vi "quiz3_valecopia.vi"() -> ()   [LabVIEW 2017]
panel:
  out "Usuarios Existentes 2":string[][](array[string])
  out "Leer 2":string[][](array[string])
  out "array 2":string[][](array[string])
  out "Tamaño users 2":i32
  out "Tab Control 2":enum32{"Page 1", "Page 2", "Page 3"}(tab)
  in  "Ingresar 2":bool
  in  "Usuario 2":string
  in  "Contraseña  2":string
  in  "Regresar 3":bool
  in  "ver usuarios 2":bool
  in  "Borrar usuario 2":string
  in  "Eliminar 2":bool
  in  "Agregar 2":bool
  in  "Contraseña usuario 2":string
  in  "nuevo usuario 2":string
  in  "Regresar 4":bool
  out "Leer":string[][](array[string])
  out "Usuarios Existentes":string[][](array[string])
  out "Tamaño users":i32
  out "array":string[][](array[string])
  out "Tab Control":enum32{"Page 1", "Page 2", "Page 3"}(tab)
  in  "Ingresar":bool
  in  "Usuario":string
  in  "Contraseña":string
  in  "Regresar":bool
  in  "ver usuarios":bool
  in  "Borrar usuario":string
  in  "Eliminar":bool
  in  "Agregar":bool
  in  "Contraseña usuario":string
  in  "nuevo usuario":string
  in  "Regresar 2":bool
  # "HOLIII..!"
  # "HOLIII..!"
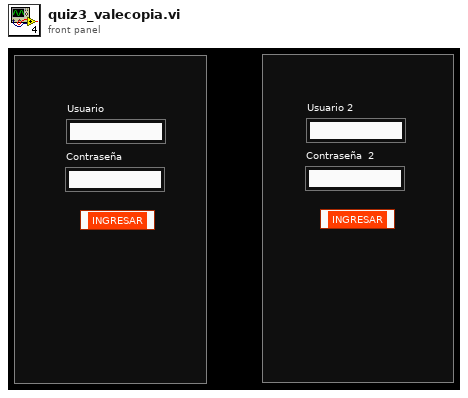
[diagram p1: front panel]
types:
  T1 = enum16{"open", "replace", "create", "open or create", "replace or create", "replace or create with confirmation"}
  T2 = typedef "Semaphore RefNum" = refnum<k1>
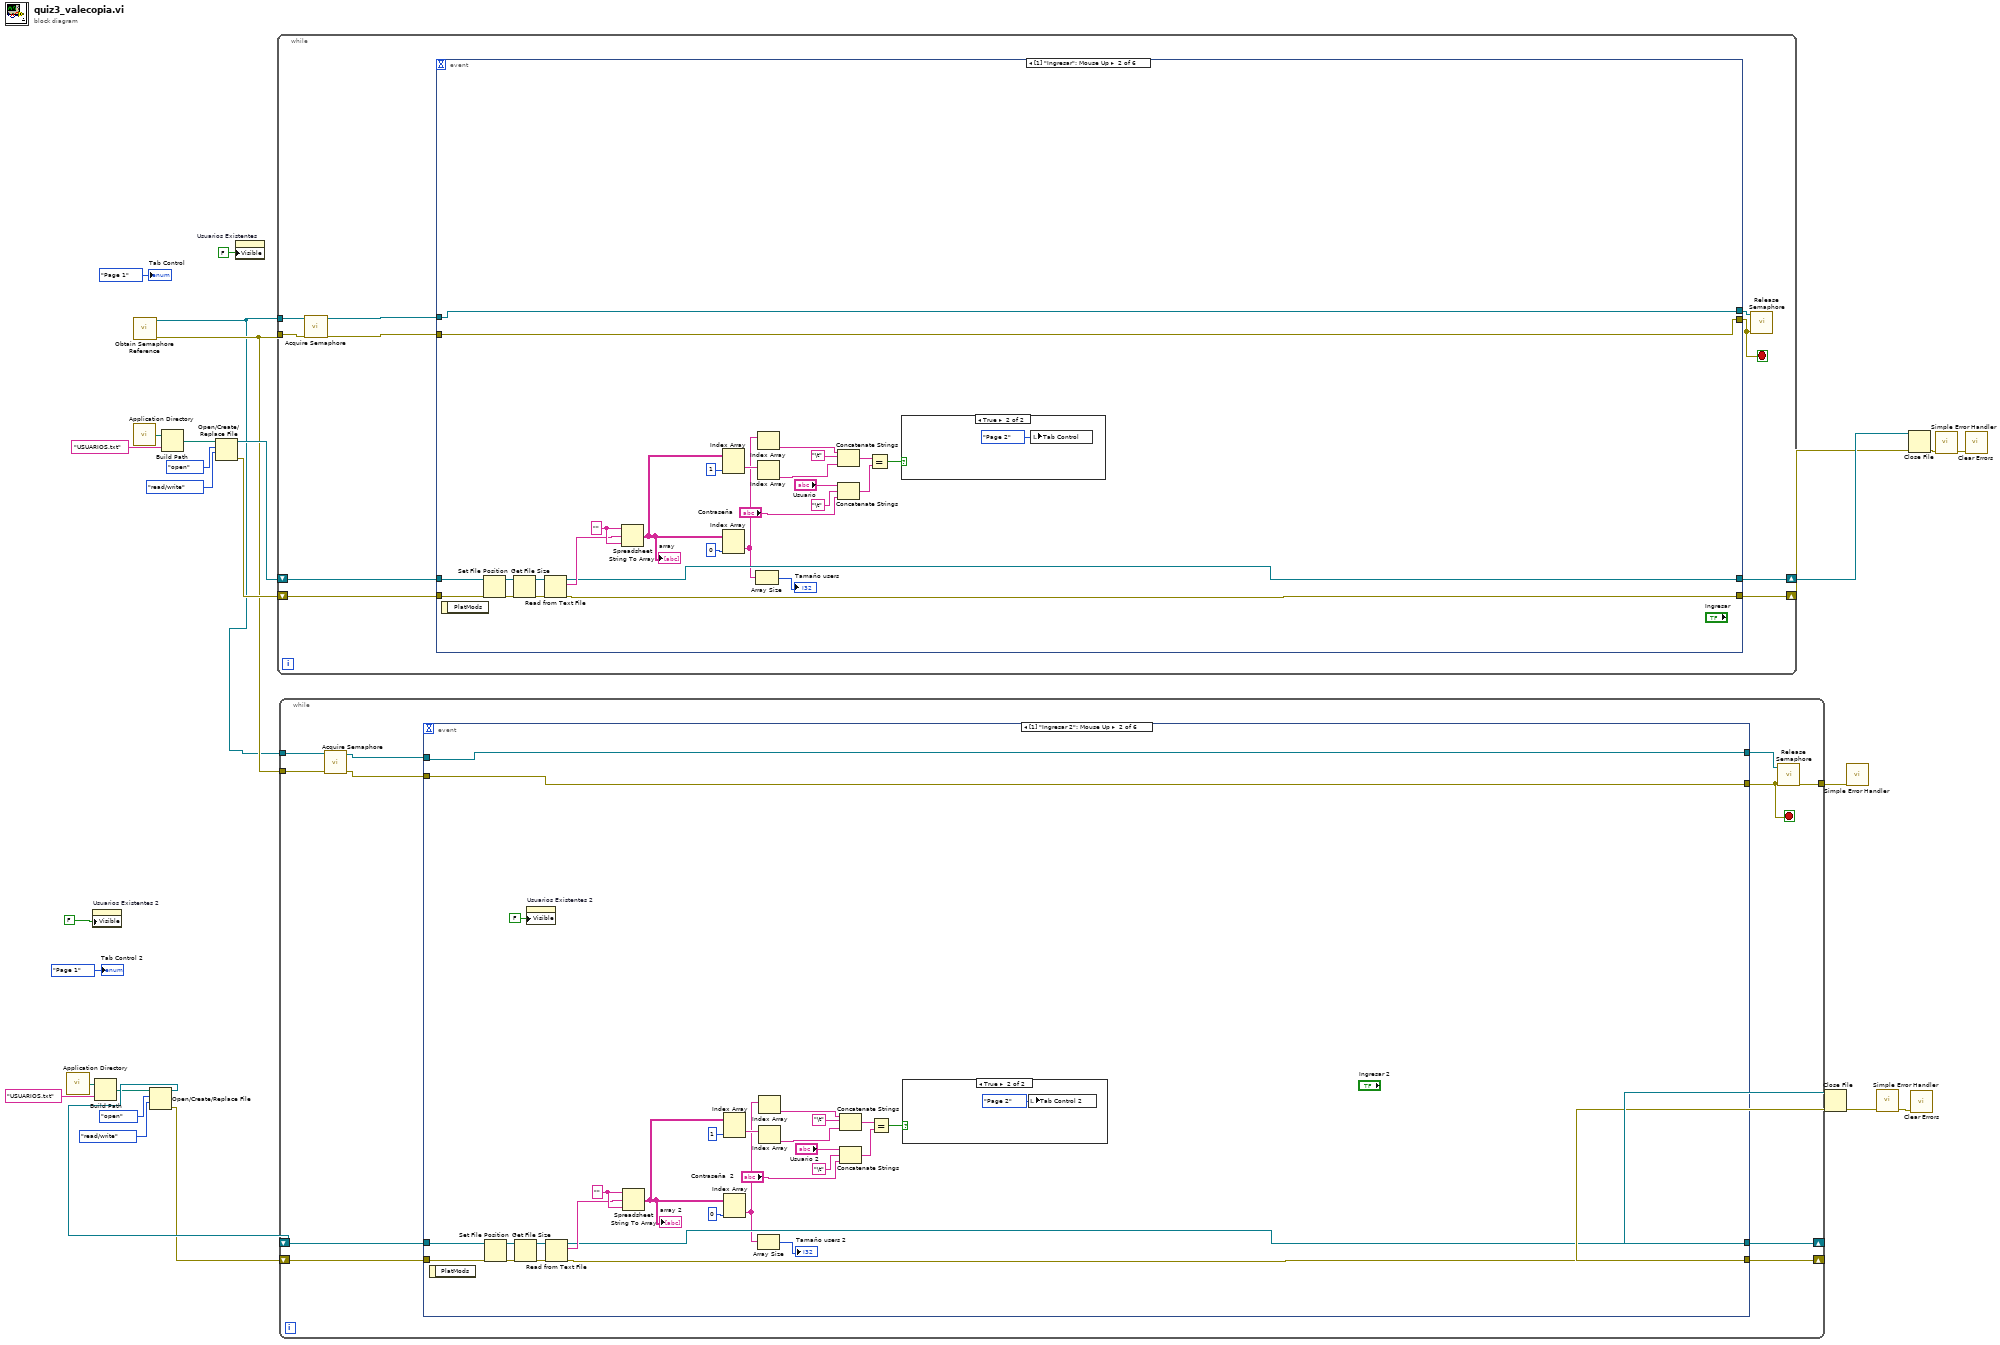
[diagram p0: block diagram]
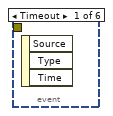
[diagram p2: hidden frame]
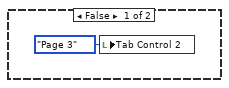
[diagram p3: hidden frame]
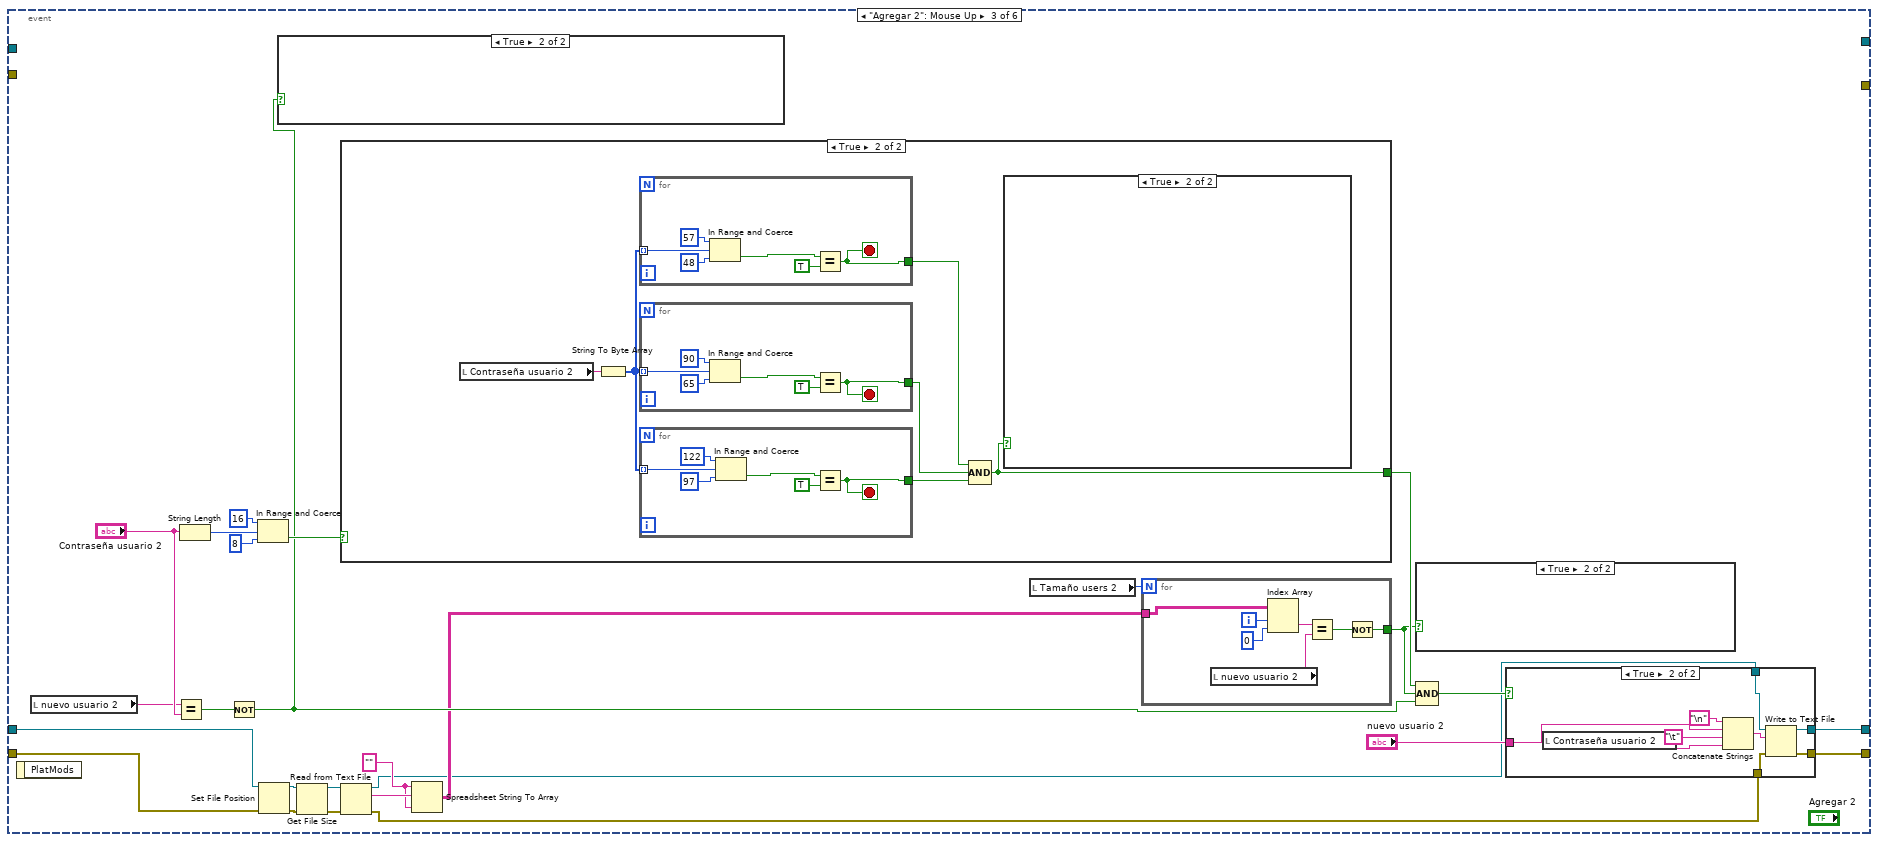
[diagram p4: hidden frame]
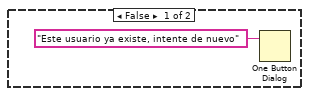
[diagram p5: hidden frame]
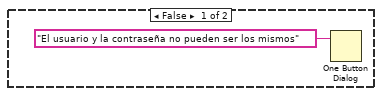
[diagram p6: hidden frame]
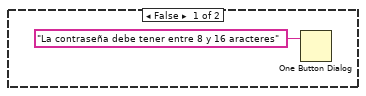
[diagram p8: hidden frame]
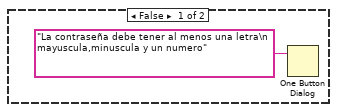
[diagram p9: hidden frame]
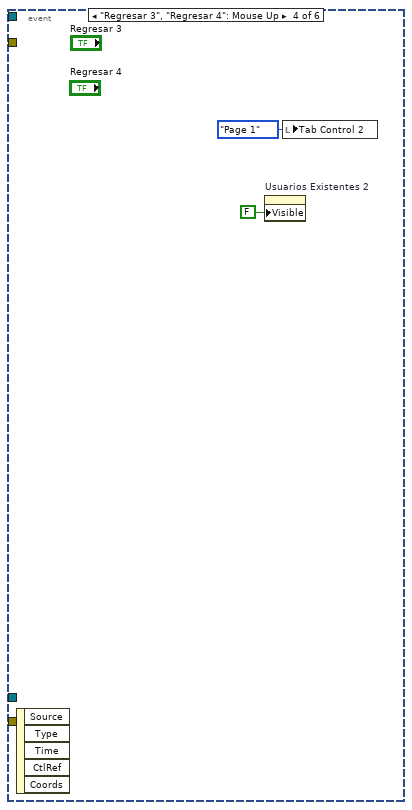
[diagram p10: hidden frame]
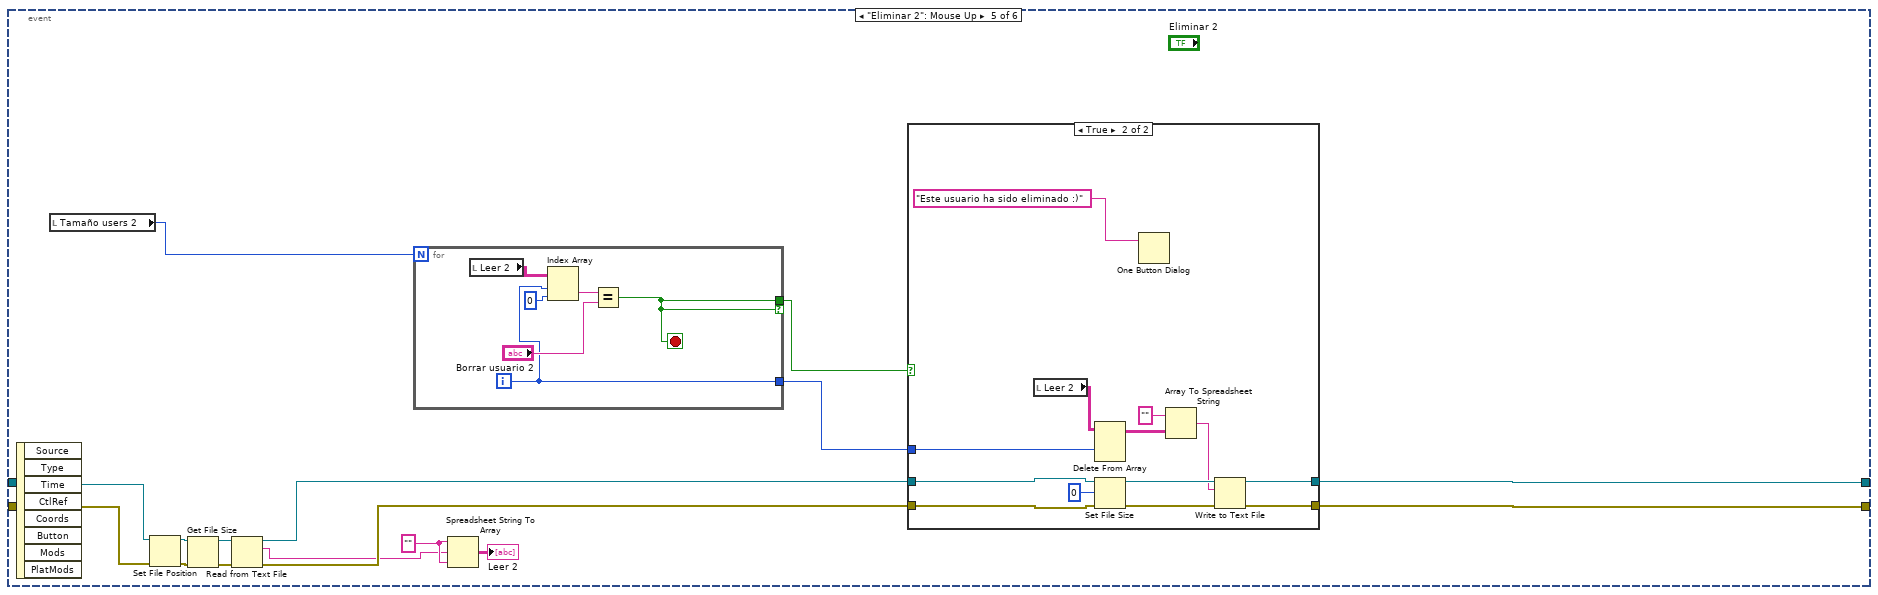
[diagram p11: hidden frame]
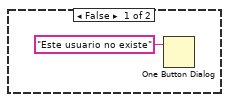
[diagram p12: hidden frame]
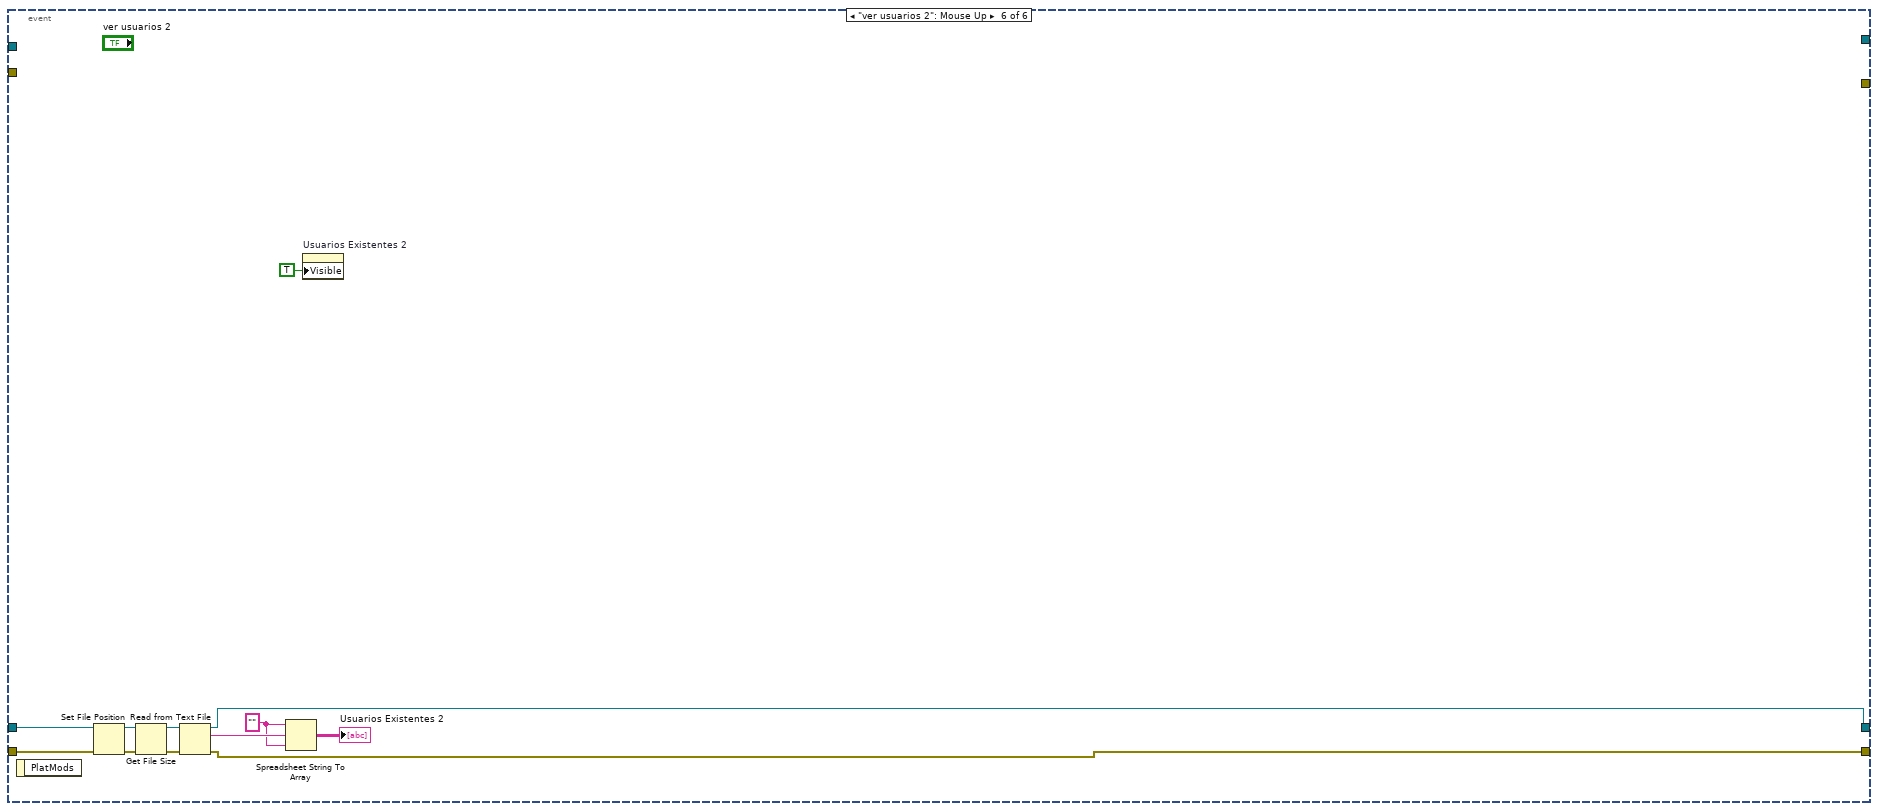
[diagram p13: hidden frame]
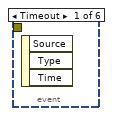
[diagram p14: hidden frame]
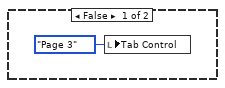
[diagram p15: hidden frame]
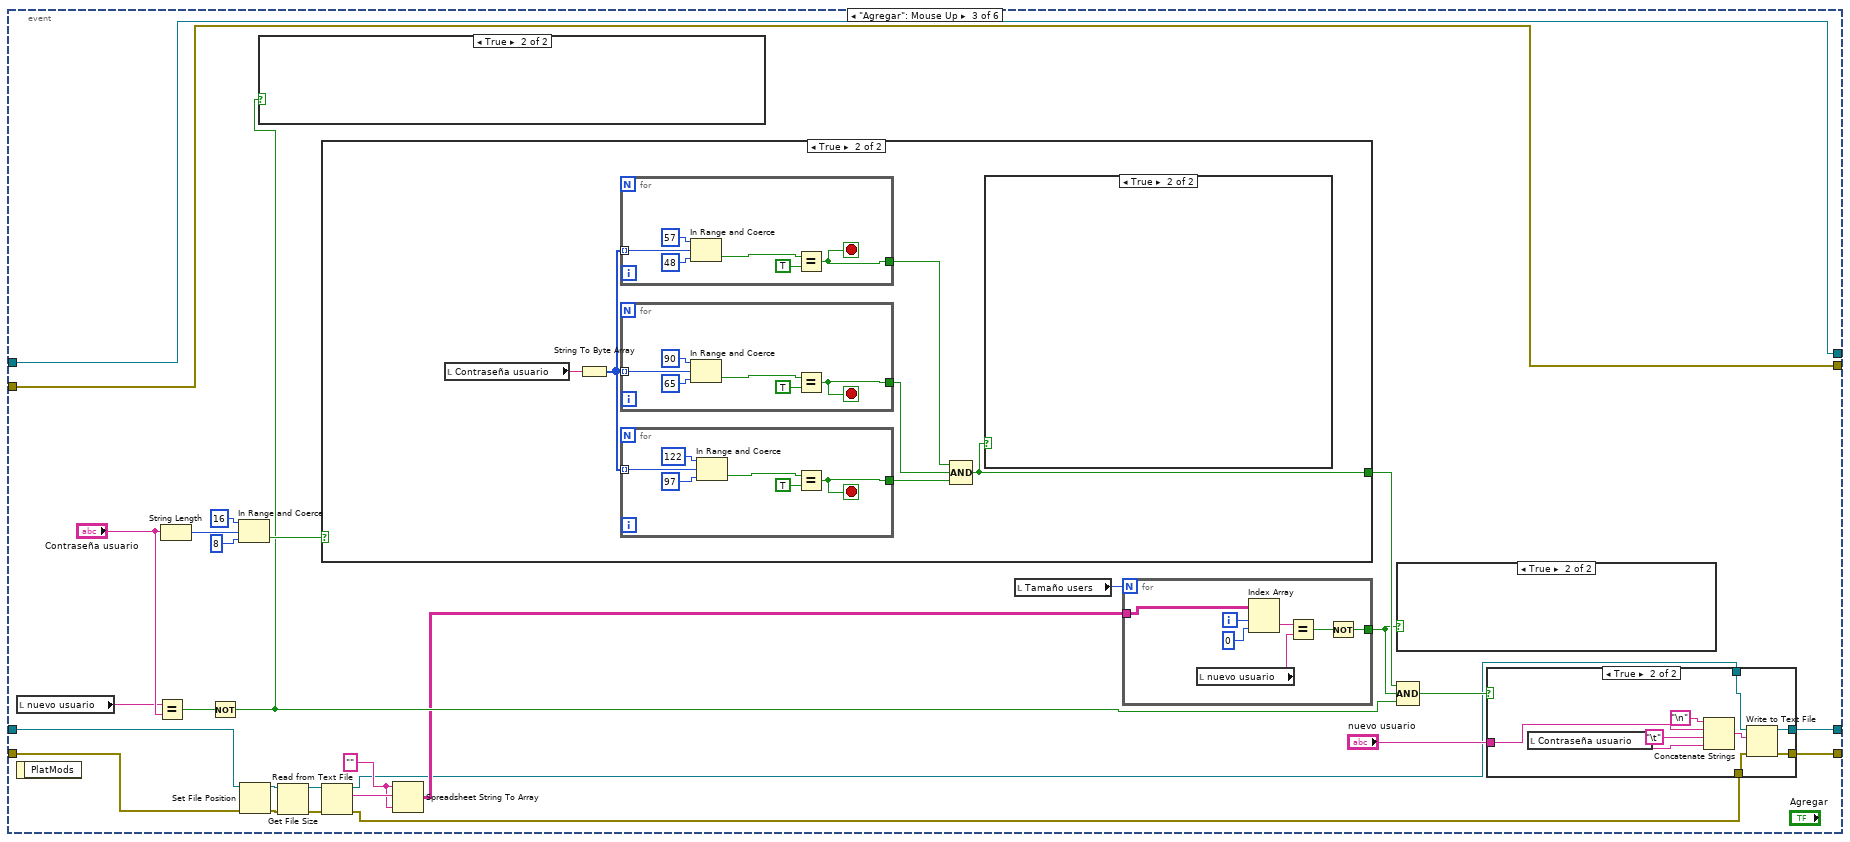
[diagram p16: hidden frame]
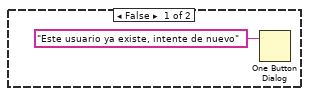
[diagram p17: hidden frame]
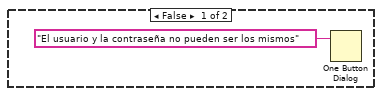
[diagram p18: hidden frame]
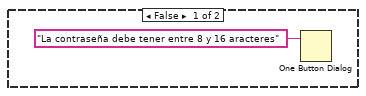
[diagram p20: hidden frame]
diagram:
  n1 = call <vilib>:"Application Directory.vi"() -> ("Application Directory"=w14:path)
  n2 = property on="Usuarios Existentes 2" class="Arr (strict)"("Visible"=FALSE) -> ()  [unwired: 2 in, 2 out]
  n3 = Build Path(base path=w14, name or relative path="USUARIOS.txt") -> (appended path=w13:path)
  n4 = call <vilib>:"Application Directory.vi"() -> ("Application Directory"=w27:path)
  n5 = call <vilib>:"Obtain Semaphore Reference.vi"() -> ("error out"=w2:errorcluster, "semaphore"=w1:T2)  [unwired: 5 in, 1 out]
  n6 = Open/Create/Replace File(file path (use dialog)=w13, operation (0:open)=T1."open", access (0:read/write)=enum16{"read/write", "read-only", "write-only"}."read/write") -> (refnum out=w17:refnum<file>, error out=w16:errorcluster)  [unwired: 3 in, 1 out]
  n7 = Build Path(base path=w27, name or relative path="USUARIOS.txt") -> (appended path=w26:path)
  n8 = Open/Create/Replace File(file path (use dialog)=w26, operation (0:open)=T1."open", access (0:read/write)=enum16{"read/write", "read-only", "write-only"}."read/write") -> (refnum out=w29:refnum<file>, error out=w4:errorcluster)  [unwired: 3 in, 1 out]
  n9 = property on="Usuarios Existentes" class="Arr (strict)"("Visible"=FALSE) -> ()  [unwired: 2 in, 2 out]
  n10 = while {
    shift-right: [w37] -> w23
    shift-left: w29 -> [w39]
    shift-right: [w38] -> w22
    shift-left: w4 -> [w36]
    tunnel: w1 -> [w34]
    tunnel: w2 -> [w32]
    stop <- w30 stop-if-true
    n11 = call <vilib>:"Acquire Semaphore.vi"("error in (no error)"=w32, "semaphore"=w34) -> ("error out"=w31:errorcluster, "semaphore out"=w33:T2)  [unwired: 3 in, 1 out]
    n12 = event shown="[1] \"Ingresar\": Mouse Up" {
      selector: _ -> [_ _ _ _ _ _]
      dyn-events: _ -> [_ _ _ _ _ _]
      timeout: _ -> [_ _ _ _ _ _]
      tunnel: w36 -> [_ w66 w77 _ w152 w189]
      tunnel: w39 -> [_ w63 w76 _ w153 w190]
      tunnel: [_ w52 w90 _ w158 w184] -> w37
      tunnel: [_ w51 w91 _ w159 w185] -> w38
      tunnel: w33 -> [_ w41 w70 w142 w145 w182]
      tunnel: w31 -> [_ w40 w69 w141 w146 w181]
      tunnel: [_ w40 w69 w141 w146 w181] -> w30
      tunnel: [_ w41 w70 w142 w145 w182] -> w35
      event Timeout {
        n13 = event-data() -> ()  [unwired: 1 in, 3 out]
      }
      event "Ingresar": Mouse Up {
        w55 = "" ("format string")
        n14 = event-data() -> ()  [unwired: 1 in, 1 out]
        n15 = Set File Position(refnum=w63, error in=w66) -> (refnum out=w62:refnum<file>, error out=w65:errorcluster)  [unwired: 2 in]
        n16 = Get File Size(file=w62, error in=w65) -> (refnum out=w61:refnum<file>, 0:w64:errorcluster)  [unwired: 1 out]
        n17 = Read from Text File(file (use dialog)=w61, error in=w64) -> (refnum out=w52:refnum<file>, text=w54:string, error out=w51:errorcluster)  [unwired: 2 in, 1 out]
        n18 = Spreadsheet String To Array(format string=w55, spreadsheet string=w54, array type (2D Dbl)=w55) -> (array=w48:string[][])  [unwired: 1 in]
        "array" <- w48
        n19 = Index Array(array=w48, index (col)=1 ("disabled index (col)")) -> (element=w53:string[])  [unwired: 1 in]
        n20 = Index Array(array=w48, index (col)=0 ("disabled index (col)")) -> (element=w47:string[])  [unwired: 1 in]
        n21 = Array Size(array=w47) -> (size(s)=→"Tamaño users":i32)
        n22 = Index Array(array=w47) -> (element=w42:string)  [unwired: 1 in]
        n23 = Index Array(array=w53) -> (element=w43:string)  [unwired: 1 in]
        n24 = Concatenate Strings(w42, "\t", w43) -> (w50:string)
        n25 = Concatenate Strings("Usuario", "\t", "Contraseña") -> (w49:string)
        n26 = Equal?(x=w50, y=w49) -> (x = y?=w45:bool)
        n27 = case shown="True" w45 {
          frame False {
            n28 = local write "Tab Control"(enum32{"Page 1", "Page 2", "Page 3"}."Page 3" ("Tab Control")) -> ()
          }
          frame True {
            n29 = local write "Tab Control"(enum32{"Page 1", "Page 2", "Page 3"}."Page 2" ("Tab Control")) -> ()
          }
        }
      }
      event "Agregar": Mouse Up {
        w74 = "" ("format string")
        n30 = local read "nuevo usuario"() -> (w84:string)
        n31 = event-data() -> ()  [unwired: 1 in, 1 out]
        n32 = Equal?(x=w84, y="Contraseña usuario") -> (x = y?=w86:bool)
        n33 = String Length(string="Contraseña usuario") -> (length=w96:i32)
        n34 = Not(x=w86) -> (.not. x?=w85:bool)
        n35 = In Range and Coerce(upper limit=16, x=w96, lower limit=8) -> (In Range?=w93:bool)  [unwired: 1 out]
        n36 = Set File Position(refnum=w76, error in=w77) -> (refnum out=w80:refnum<file>, error out=w78:errorcluster)  [unwired: 2 in]
        n37 = case shown="True" w85 {
          frame False {
            n38 = One Button Dialog(message="El usuario y la contraseña no pueden ser los mismos") -> ()  [unwired: 1 in, 1 out]
          }
          frame True {
          }
        }
        n39 = Get File Size(file=w80, error in=w78) -> (refnum out=w81:refnum<file>, 0:w79:errorcluster)  [unwired: 1 out]
        n40 = case shown="True" w93 {
          tunnel: [_ w116] -> w87
          frame False {
            n41 = One Button Dialog(message="La contraseña debe tener entre 8 y 16 aracteres") -> ()  [unwired: 1 in, 1 out]
          }
          frame True {
            n42 = local read "Contraseña usuario"() -> (w121:string)
            n43 = String To Byte Array(string=w121) -> (unsigned byte array=w119:u8[])
            n44 = for {
              tunnel: w119 -> [w129] mode=indexing
              tunnel: [w128] -> w120
              stop <- w128 stop-if-true
              n45 = In Range and Coerce(upper limit=u8 57, x=w129, lower limit=u8 48) -> (In Range?=w131:bool)  [unwired: 1 out]
              n46 = Equal?(x=w131, y=TRUE) -> (x = y?=w128:bool)
            }
            n47 = for {
              tunnel: w119 -> [w125] mode=indexing
              tunnel: [w122] -> w118
              stop <- w122 stop-if-true
              n48 = In Range and Coerce(upper limit=u8 90, x=w125, lower limit=u8 65) -> (In Range?=w124:bool)  [unwired: 1 out]
              n49 = Equal?(x=w124, y=TRUE) -> (x = y?=w122:bool)
            }
            n50 = for {
              tunnel: w119 -> [w135] mode=indexing
              tunnel: [w136] -> w117
              stop <- w136 stop-if-true
              n51 = In Range and Coerce(upper limit=u8 122, x=w135, lower limit=u8 97) -> (In Range?=w138:bool)  [unwired: 1 out]
              n52 = Equal?(x=w138, y=TRUE) -> (x = y?=w136:bool)
            }
            n53 = Compound Arithmetic op=AND(w120, w118, w117) -> (w116:bool)
            n54 = case shown="True" w116 {
              frame False {
                n55 = One Button Dialog(message="La contraseña debe tener al menos una letra\n mayuscula,minuscula y un numero") -> ()  [unwired: 1 in, 1 out]
              }
              frame True {
              }
            }
          }
        }
        n56 = Read from Text File(file (use dialog)=w81, error in=w79) -> (refnum out=w71:refnum<file>, text=w75:string, error out=w72:errorcluster)  [unwired: 2 in, 1 out]
        n57 = Spreadsheet String To Array(format string=w74, spreadsheet string=w75, array type (2D Dbl)=w74) -> (array=w73:string[][])  [unwired: 1 in]
        n58 = local read "Tamaño users"() -> (w92:i32)
        n59 = for {
          N: w92 -> [_]
          tunnel: [w100] -> w82
          tunnel: w73 -> [w99]
          i -> [w104]
          n60 = local read "nuevo usuario"() -> (w102:string)
          n61 = Index Array(array=w99, index (row)=w104, index (col)=0 ("disabled index (col)")) -> (element=w103:string)
          n62 = Equal?(x=w103, y=w102) -> (x = y?=w101:bool)
          n63 = Not(x=w101) -> (.not. x?=w100:bool)
        }
        n64 = case shown="True" w82 {
          frame False {
            n65 = One Button Dialog(message="Este usuario ya existe, intente de nuevo") -> ()  [unwired: 1 in, 1 out]
          }
          frame True {
          }
        }
        n66 = Compound Arithmetic op=AND(w87, w82, w85) -> (w88:bool)
        n67 = case shown="True" w88 {
          tunnel: [_ w110] -> w90
          tunnel: [_ w109] -> w91
          tunnel: "nuevo usuario" -> [_ w108]
          tunnel: w71 -> [_ w107]
          tunnel: w72 -> [_ w106]
          frame False {
          }
          frame True {
            n68 = local read "Contraseña usuario"() -> (w111:string)
            n69 = Concatenate Strings("\n", w108, "\t", w111) -> (w112:string)
            n70 = Write to Text File(file (use dialog)=w107, text=w112, error in=w106) -> (refnum out=w110:refnum<file>, error out=w109:errorcluster)  [unwired: 1 in, 1 out]
          }
        }
      }
      event "Regresar", "Regresar 2": Mouse Up {
        n71 = event-data() -> ()  [unwired: 1 in, 5 out]
        n72 = property on="Usuarios Existentes" class="Arr (strict)"("Visible"=FALSE) -> ()  [unwired: 2 in, 2 out]
        n73 = local write "Tab Control"(enum32{"Page 1", "Page 2", "Page 3"}."Page 1" ("Tab Control")) -> ()
      }
      event "Eliminar": Mouse Up {
        w150 = "" ("format string")
        n74 = event-data() -> ()  [unwired: 1 in, 1 out]
        n75 = local read "Tamaño users"() -> (w161:i32)
        n76 = Set File Position(refnum=w153, error in=w152) -> (refnum out=w156:refnum<file>, error out=w154:errorcluster)  [unwired: 2 in]
        n77 = Get File Size(file=w156, error in=w154) -> (refnum out=w157:refnum<file>, 0:w155:errorcluster)  [unwired: 1 out]
        n78 = Read from Text File(file (use dialog)=w157, error in=w155) -> (refnum out=w151:refnum<file>, text=w149:string)  [unwired: 2 in, 2 out]
        n79 = for {
          N: w161 -> [_]
          tunnel: [w178] -> w160
          tunnel: [w175] -> w147 if=w175
          i -> [w178]
          stop <- w175 stop-if-true
          n80 = local read "Leer"() -> (w177:string[][])
          n81 = Index Array "Index Array"(array=w177, index (row)=w178, index (col)=0 ("disabled index (col)")) -> (element=w176:string)
          n82 = Equal?(x=w176, y="Borrar usuario") -> (x = y?=w175:bool)
        }
        n83 = Spreadsheet String To Array(format string=w150, spreadsheet string=w149, array type (2D Dbl)=w150) -> (array=→"Leer":string[][])  [unwired: 1 in]
        n84 = case shown="True" w147 {
          tunnel: w160 -> [_ w174]
          tunnel: w151 -> [_ w170]
          tunnel: [_ w168] -> w159
          tunnel: [_ w167] -> w158
          frame False {
            n85 = One Button Dialog(message="Este usuario no existe") -> ()  [unwired: 1 in, 1 out]
          }
          frame True {
            n86 = local read "Leer"() -> (w165:string[][])
            n87 = Delete From Array "Delete From Array"(array=w165, index (row)=w174) -> (array with subset deleted=w164:string[][])  [unwired: 2 in, 1 out]
            n88 = Set File Size(6:i64 0 ("size (in bytes)"), 7:w170) -> (0:w169:errorcluster, 3:w172:refnum<file>)  [unwired: 1 in]
            n89 = One Button Dialog(message="Este usuario ha sido eliminado :)") -> ()  [unwired: 1 in, 1 out]
            n90 = Array To Spreadsheet String(array=w164, 3:"" ("format string")) -> (spreadsheet string=w171:string)  [unwired: 1 in]
            n91 = Write to Text File(file (use dialog)=w172, text=w171, error in=w169) -> (refnum out=w167:refnum<file>, error out=w168:errorcluster)  [unwired: 1 in, 1 out]
          }
        }
      }
      event "ver usuarios": Mouse Up {
        w187 = "" ("format string")
        n92 = event-data() -> ()  [unwired: 1 in, 1 out]
        n93 = Set File Position(refnum=w190, error in=w189) -> (refnum out=w193:refnum<file>, error out=w191:errorcluster)  [unwired: 2 in]
        n94 = Get File Size(file=w193, error in=w191) -> (refnum out=w194:refnum<file>, 0:w192:errorcluster)  [unwired: 1 out]
        n95 = Read from Text File(file (use dialog)=w194, error in=w192) -> (refnum out=w184:refnum<file>, text=w188:string, error out=w185:errorcluster)  [unwired: 2 in, 1 out]
        n96 = Spreadsheet String To Array(format string=w187, spreadsheet string=w188, array type (2D Dbl)=w187) -> (array=→"Usuarios Existentes":string[][])  [unwired: 1 in]
        n97 = property on="Usuarios Existentes" class="Arr (strict)"("Visible"=TRUE) -> ()  [unwired: 2 in, 2 out]
      }
    }
    n98 = call <vilib>:"Release Semaphore.vi"("error in (no error)"=w30, "semaphore"=w35) -> ()  [unwired: 4 in, 2 out]
  }
  n99 = while {
    shift-right: [w203] -> w10
    shift-left: w17 -> [w205]
    shift-right: [w204] -> w9
    shift-left: w16 -> [w200]
    tunnel: w1 -> [w202]
    tunnel: w2 -> [w199]
    tunnel: [w195] -> w3
    stop <- w196 stop-if-true
    n100 = call <vilib>:"Acquire Semaphore.vi"("error in (no error)"=w199, "semaphore"=w202) -> ("error out"=w198:errorcluster, "semaphore out"=w201:T2)  [unwired: 3 in, 1 out]
    n101 = event shown="[1] \"Ingresar 2\": Mouse Up" {
      selector: _ -> [_ _ _ _ _ _]
      dyn-events: _ -> [_ _ _ _ _ _]
      timeout: _ -> [_ _ _ _ _ _]
      tunnel: w200 -> [_ w233 w242 _ w314 w350]
      tunnel: w205 -> [_ w230 w241 _ w315 w351]
      tunnel: [_ w219 w255 _ w320 w345] -> w203
      tunnel: [_ w218 w256 _ w321 w346] -> w204
      tunnel: w201 -> [_ w207 _ _ _ _]
      tunnel: w198 -> [_ w206 _ _ _ _]
      tunnel: [_ w206 _ _ _ _] -> w196
      tunnel: [_ w207 _ _ _ _] -> w197
      event Timeout {
        n102 = event-data() -> ()  [unwired: 1 in, 3 out]
      }
      event "Ingresar 2": Mouse Up {
        w222 = "" ("format string")
        n103 = event-data() -> ()  [unwired: 1 in, 1 out]
        n104 = Set File Position(refnum=w230, error in=w233) -> (refnum out=w229:refnum<file>, error out=w232:errorcluster)  [unwired: 2 in]
        n105 = Get File Size(file=w229, error in=w232) -> (refnum out=w228:refnum<file>, 0:w231:errorcluster)  [unwired: 1 out]
        n106 = property on="Usuarios Existentes 2" class="Arr (strict)"("Visible"=FALSE) -> ()  [unwired: 2 in, 2 out]
        n107 = Read from Text File(file (use dialog)=w228, error in=w231) -> (refnum out=w219:refnum<file>, text=w221:string, error out=w218:errorcluster)  [unwired: 2 in, 1 out]
        n108 = Spreadsheet String To Array(format string=w222, spreadsheet string=w221, array type (2D Dbl)=w222) -> (array=w215:string[][])  [unwired: 1 in]
        "array 2" <- w215
        n109 = Index Array(array=w215, index (col)=1 ("disabled index (col)")) -> (element=w220:string[])  [unwired: 1 in]
        n110 = Index Array(array=w215, index (col)=0 ("disabled index (col)")) -> (element=w214:string[])  [unwired: 1 in]
        n111 = Array Size(array=w214) -> (size(s)=→"Tamaño users 2":i32)
        n112 = Index Array(array=w214) -> (element=w209:string)  [unwired: 1 in]
        n113 = Index Array(array=w220) -> (element=w210:string)  [unwired: 1 in]
        n114 = Concatenate Strings(w209, "\t", w210) -> (w217:string)
        n115 = Concatenate Strings("Usuario 2", "\t", "Contraseña  2") -> (w216:string)
        n116 = Equal?(x=w217, y=w216) -> (x = y?=w212:bool)
        n117 = case shown="True" w212 {
          frame False {
            n118 = local write "Tab Control 2"(enum32{"Page 1", "Page 2", "Page 3"}."Page 3" ("Tab Control")) -> ()
          }
          frame True {
            n119 = local write "Tab Control 2"(enum32{"Page 1", "Page 2", "Page 3"}."Page 2" ("Tab Control")) -> ()
          }
        }
      }
      event "Agregar 2": Mouse Up {
        w239 = "" ("format string")
        n120 = event-data() -> ()  [unwired: 1 in, 1 out]
        n121 = local read "nuevo usuario 2"() -> (w249:string)
        n122 = Equal?(x=w249, y="Contraseña usuario 2") -> (x = y?=w251:bool)
        n123 = String Length(string="Contraseña usuario 2") -> (length=w261:i32)
        n124 = Not(x=w251) -> (.not. x?=w250:bool)
        n125 = In Range and Coerce(upper limit=16, x=w261, lower limit=8) -> (In Range?=w258:bool)  [unwired: 1 out]
        n126 = Set File Position(refnum=w241, error in=w242) -> (refnum out=w245:refnum<file>, error out=w243:errorcluster)  [unwired: 2 in]
        n127 = case shown="True" w250 {
          frame False {
            n128 = One Button Dialog(message="El usuario y la contraseña no pueden ser los mismos") -> ()  [unwired: 1 in, 1 out]
          }
          frame True {
          }
        }
        n129 = Get File Size(file=w245, error in=w243) -> (refnum out=w246:refnum<file>, 0:w244:errorcluster)  [unwired: 1 out]
        n130 = case shown="True" w258 {
          tunnel: [_ w281] -> w252
          frame False {
            n131 = One Button Dialog(message="La contraseña debe tener entre 8 y 16 aracteres") -> ()  [unwired: 1 in, 1 out]
          }
          frame True {
            n132 = local read "Contraseña usuario 2"() -> (w286:string)
            n133 = String To Byte Array(string=w286) -> (unsigned byte array=w284:u8[])
            n134 = for {
              tunnel: w284 -> [w294] mode=indexing
              tunnel: [w293] -> w285
              stop <- w293 stop-if-true
              n135 = In Range and Coerce(upper limit=u8 57, x=w294, lower limit=u8 48) -> (In Range?=w296:bool)  [unwired: 1 out]
              n136 = Equal?(x=w296, y=TRUE) -> (x = y?=w293:bool)
            }
            n137 = for {
              tunnel: w284 -> [w290] mode=indexing
              tunnel: [w287] -> w283
              stop <- w287 stop-if-true
              n138 = In Range and Coerce(upper limit=u8 90, x=w290, lower limit=u8 65) -> (In Range?=w289:bool)  [unwired: 1 out]
              n139 = Equal?(x=w289, y=TRUE) -> (x = y?=w287:bool)
            }
            n140 = for {
              tunnel: w284 -> [w300] mode=indexing
              tunnel: [w301] -> w282
              stop <- w301 stop-if-true
              n141 = In Range and Coerce(upper limit=u8 122, x=w300, lower limit=u8 97) -> (In Range?=w303:bool)  [unwired: 1 out]
              n142 = Equal?(x=w303, y=TRUE) -> (x = y?=w301:bool)
            }
            n143 = Compound Arithmetic op=AND(w285, w283, w282) -> (w281:bool)
            n144 = case shown="True" w281 {
              frame False {
                n145 = One Button Dialog(message="La contraseña debe tener al menos una letra\n mayuscula,minuscula y un numero") -> ()  [unwired: 1 in, 1 out]
              }
              frame True {
              }
            }
          }
        }
        n146 = Read from Text File(file (use dialog)=w246, error in=w244) -> (refnum out=w236:refnum<file>, text=w240:string, error out=w237:errorcluster)  [unwired: 2 in, 1 out]
        n147 = Spreadsheet String To Array(format string=w239, spreadsheet string=w240, array type (2D Dbl)=w239) -> (array=w238:string[][])  [unwired: 1 in]
        n148 = local read "Tamaño users 2"() -> (w257:i32)
        n149 = for {
          N: w257 -> [_]
          tunnel: [w265] -> w247
          tunnel: w238 -> [w264]
          i -> [w269]
          n150 = local read "nuevo usuario 2"() -> (w267:string)
          n151 = Index Array(array=w264, index (row)=w269, index (col)=0 ("disabled index (col)")) -> (element=w268:string)
          n152 = Equal?(x=w268, y=w267) -> (x = y?=w266:bool)
          n153 = Not(x=w266) -> (.not. x?=w265:bool)
        }
        n154 = case shown="True" w247 {
          frame False {
            n155 = One Button Dialog(message="Este usuario ya existe, intente de nuevo") -> ()  [unwired: 1 in, 1 out]
          }
          frame True {
          }
        }
        n156 = Compound Arithmetic op=AND(w252, w247, w250) -> (w253:bool)
        n157 = case shown="True" w253 {
          tunnel: [_ w275] -> w255
          tunnel: [_ w274] -> w256
          tunnel: "nuevo usuario 2" -> [_ w273]
          tunnel: w236 -> [_ w272]
          tunnel: w237 -> [_ w271]
          frame False {
          }
          frame True {
            n158 = local read "Contraseña usuario 2"() -> (w276:string)
            n159 = Concatenate Strings("\n", w273, "\t", w276) -> (w277:string)
            n160 = Write to Text File(file (use dialog)=w272, text=w277, error in=w271) -> (refnum out=w275:refnum<file>, error out=w274:errorcluster)  [unwired: 1 in, 1 out]
          }
        }
      }
      event "Regresar 3", "Regresar 4": Mouse Up {
        n161 = event-data() -> ()  [unwired: 1 in, 5 out]
        n162 = property on="Usuarios Existentes 2" class="Arr (strict)"("Visible"=FALSE) -> ()  [unwired: 2 in, 2 out]
        n163 = local write "Tab Control 2"(enum32{"Page 1", "Page 2", "Page 3"}."Page 1" ("Tab Control")) -> ()
      }
      event "Eliminar 2": Mouse Up {
        w311 = "" ("format string")
        n164 = event-data() -> ()  [unwired: 1 in, 8 out]
        n165 = local read "Tamaño users 2"() -> (w323:i32)
        n166 = Set File Position(refnum=w315, error in=w314) -> (refnum out=w318:refnum<file>, error out=w316:errorcluster)  [unwired: 2 in]
        n167 = Get File Size(file=w318, error in=w316) -> (refnum out=w319:refnum<file>, 0:w317:errorcluster)  [unwired: 1 out]
        n168 = Read from Text File(file (use dialog)=w319, error in=w317) -> (refnum out=w313:refnum<file>, text=w310:string, error out=w312:errorcluster)  [unwired: 2 in, 1 out]
        n169 = for {
          N: w323 -> [_]
          tunnel: [w341] -> w322
          tunnel: [w338] -> w308 if=w338
          i -> [w341]
          stop <- w338 stop-if-true
          n170 = local read "Leer 2"() -> (w340:string[][])
          n171 = Index Array "Index Array"(array=w340, index (row)=w341, index (col)=0 ("disabled index (col)")) -> (element=w339:string)
          n172 = Equal?(x=w339, y="Borrar usuario 2") -> (x = y?=w338:bool)
        }
        n173 = Spreadsheet String To Array(format string=w311, spreadsheet string=w310, array type (2D Dbl)=w311) -> (array=→"Leer 2":string[][])  [unwired: 1 in]
        n174 = case shown="True" w308 {
          tunnel: w322 -> [_ w337]
          tunnel: w313 -> [_ w333]
          tunnel: w312 -> [_ w332]
          tunnel: [_ w330] -> w321
          tunnel: [_ w329] -> w320
          frame False {
            n175 = One Button Dialog(message="Este usuario no existe") -> ()  [unwired: 1 in, 1 out]
          }
          frame True {
            n176 = local read "Leer 2"() -> (w327:string[][])
            n177 = Delete From Array "Delete From Array"(array=w327, index (row)=w337) -> (array with subset deleted=w326:string[][])  [unwired: 2 in, 1 out]
            n178 = Set File Size(4:w332, 6:i64 0 ("size (in bytes)"), 7:w333) -> (0:w331:errorcluster, 3:w335:refnum<file>)
            n179 = One Button Dialog(message="Este usuario ha sido eliminado :)") -> ()  [unwired: 1 in, 1 out]
            n180 = Array To Spreadsheet String(array=w326, 3:"" ("format string")) -> (spreadsheet string=w334:string)  [unwired: 1 in]
            n181 = Write to Text File(file (use dialog)=w335, text=w334, error in=w331) -> (refnum out=w329:refnum<file>, error out=w330:errorcluster)  [unwired: 1 in, 1 out]
          }
        }
      }
      event "ver usuarios 2": Mouse Up {
        w348 = "" ("format string")
        n182 = event-data() -> ()  [unwired: 1 in, 1 out]
        n183 = Set File Position(refnum=w351, error in=w350) -> (refnum out=w354:refnum<file>, error out=w352:errorcluster)  [unwired: 2 in]
        n184 = Get File Size(file=w354, error in=w352) -> (refnum out=w355:refnum<file>, 0:w353:errorcluster)  [unwired: 1 out]
        n185 = Read from Text File(file (use dialog)=w355, error in=w353) -> (refnum out=w345:refnum<file>, text=w349:string, error out=w346:errorcluster)  [unwired: 2 in, 1 out]
        n186 = Spreadsheet String To Array(format string=w348, spreadsheet string=w349, array type (2D Dbl)=w348) -> (array=→"Usuarios Existentes 2":string[][])  [unwired: 1 in]
        n187 = property on="Usuarios Existentes 2" class="Arr (strict)"("Visible"=TRUE) -> ()  [unwired: 2 in, 2 out]
      }
    }
    n188 = call <vilib>:"Release Semaphore.vi"("error in (no error)"=w196, "semaphore"=w197) -> ("error out"=w195:errorcluster)  [unwired: 4 in, 1 out]
  }
  n189 = Close File(refnum=w10, error in=w9) -> (error out=w8:errorcluster)  [unwired: 1 out]
  n190 = call <vilib>:"Simple Error Handler.vi"("error in (no error)"=w3) -> ()  [unwired: 4 in, 5 out]
  n191 = call <vilib>:"Simple Error Handler.vi"("error in (no error)"=w8) -> ("error out"=w7:errorcluster)  [unwired: 4 in, 4 out]
  n192 = Close File(refnum=w23, error in=w22) -> (error out=w21:errorcluster)  [unwired: 1 out]
  n193 = call <vilib>:"Clear Errors.vi"("error in (no error)"=w7) -> ()  [unwired: 5 in, 2 out]
  n194 = call <vilib>:"Simple Error Handler.vi"("error in (no error)"=w21) -> ("error out"=w20:errorcluster)  [unwired: 4 in, 4 out]
  n195 = call <vilib>:"Clear Errors.vi"("error in (no error)"=w20) -> ()  [unwired: 5 in, 2 out]
  "Tab Control" <- enum32{"Page 1", "Page 2", "Page 3"}."Page 1" ("Tab Control")
  "Tab Control 2" <- enum32{"Page 1", "Page 2", "Page 3"}."Page 1" ("Tab Control")
